vi "ZeroPigeon.vi"(9 "Pigeon":T1={"DeviceStatus"={"status"=FALSE, "code"=0, "source"=""}, "Device Number"=0, "Type"=352321536, "Device ID"=0, "Handle"=0, "UsageFrame"=0, "Library Path"=path ""} {"Type" items=["CAN"=352321536, "TalonSRX"=33554432]}) -> (3 "Pigeon":T1={"DeviceStatus"={"status"=FALSE, "code"=0, "source"=""}, "Device Number"=0, "Type"=352321536, "Device ID"=0, "Handle"=0, "UsageFrame"=0, "Library Path"=path ""} {"Type" items=["CAN"=352321536, "TalonSRX"=33554432]})   [LabVIEW 2017]
uses:
  <vilib>/Rock Robotics/WPI/ThirdParty/Phoenix-LabVIEW/Pigeon IMU/CTRE_PigeonIMU_DeviceRef.ctl
  <vilib>/Rock Robotics/WPI/ThirdParty/Phoenix-LabVIEW/Pigeon IMU/CTRE_PigeonIMU_ConnectionType.ctl
  Constants.vi
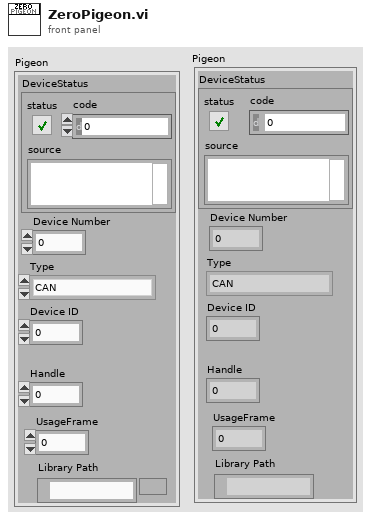
[diagram p1: front panel]
types:
  T1 = typedef "CTRE_PigeonIMU_DeviceRef.ctl" = cluster{"DeviceStatus":errorcluster, "Device Number":u8, "Type":T2, "Device ID":u32, "Handle":u64, "UsageFrame":u32, "Library Path":path}
  T2 = typedef "CTRE_PigeonIMU_ConnectionType.ctl" = u32
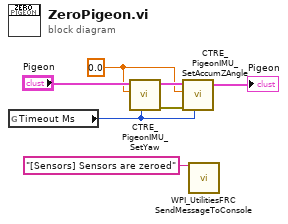
[diagram p0: block diagram]
diagram:
  w4 = 0.0 ("Value")
  n1 = global read "Constants.vi" "Timeout Ms"() -> (w1:i32)
  n2 = call <vilib>:"CTRE_PigeonIMU_SetYaw.vi"("timeoutMs"=w1, "Value"=w4, "PigeonIMUDevRef"="Pigeon") -> ("error out"=w7:errorcluster, "PigeonIMUDevRef"=w6:T1)  [unwired: 7 in]
  n3 = call <vilib>:"CTRE_PigeonIMU_SetAccumZAngle.vi"("timeoutMs"=w1, "error in (no error)"=w7, "Angle (Deg)"=w4, "PigeonIMUDevRef"=w6) -> ("PigeonIMUDevRef"=→"Pigeon":T1)  [unwired: 6 in, 1 out]
  n4 = call <vilib>:"WPI_UtilitiesFRC SendMessageToConsole.vi"("Message"="[Sensors] Sensors are zeroed") -> ()  [unwired: 14 in, 1 out]
